vi "UTILITY Bool to String.vi"(11 "Input Bool":bool) -> (3 "Output String":string)   [LabVIEW 2016]
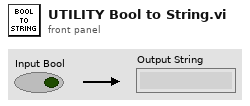
[diagram p1: front panel]
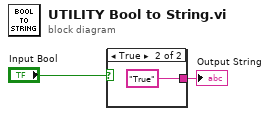
[diagram p0: block diagram]
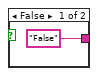
[diagram p2: hidden frame]
diagram:
  n1 = case shown="True" "Input Bool" {
    tunnel: ["False" "True"] -> w1
    frame False {
    }
    frame True {
    }
  }
  "Output String" <- w1
